vi "Trajectory_Execution_Dash_Write.vi"   [LabVIEW 2019]
uses:
  Trajectory_Execution_Globals.vi
  <vilib>/Rock Robotics/Network Tables/NT Write Number.vi
  <vilib>/Rock Robotics/Network Tables/NT Write Boolean.vi
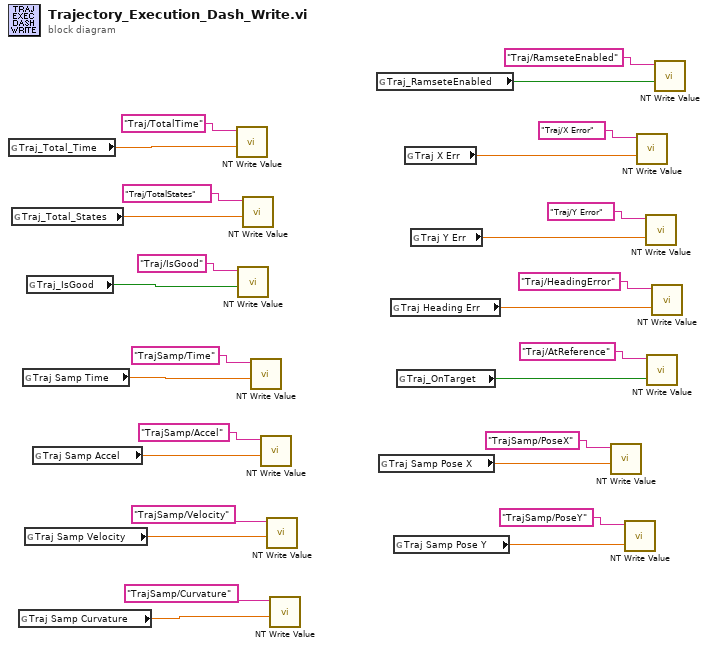
[diagram p0: block diagram]
diagram:
  n1 = global read "Trajectory_Execution_Globals.vi" "Traj_Total_Time"() -> (w14:dbl)
  n2 = global read "Trajectory_Execution_Globals.vi" "Traj_Total_States"() -> (w13:dbl)
  n3 = global read "Trajectory_Execution_Globals.vi" "Traj Samp Curvature"() -> (w8:dbl)
  n4 = global read "Trajectory_Execution_Globals.vi" "Traj Samp Time"() -> (w11:dbl)
  n5 = global read "Trajectory_Execution_Globals.vi" "Traj Samp Velocity"() -> (w9:dbl)
  n6 = global read "Trajectory_Execution_Globals.vi" "Traj_IsGood"() -> (w12:bool)
  n7 = global read "Trajectory_Execution_Globals.vi" "Traj Samp Accel"() -> (w10:dbl)
  n8 = call-poly <vilib>:"NT Write Value.vi"("Numeric"=w14, "Name"="Traj/TotalTime") -> ()  [unwired: 9 in, 1 out]
  n9 = call-poly <vilib>:"NT Write Value.vi"("Boolean"=w12, "Name"="Traj/IsGood") -> ()  [unwired: 9 in, 1 out]
  n10 = call-poly <vilib>:"NT Write Value.vi"("Numeric"=w13, "Name"="Traj/TotalStates") -> ()  [unwired: 9 in, 1 out]
  n11 = call-poly <vilib>:"NT Write Value.vi"("Numeric"=w11, "Name"="TrajSamp/Time") -> ()  [unwired: 9 in, 1 out]
  n12 = call-poly <vilib>:"NT Write Value.vi"("Numeric"=w10, "Name"="TrajSamp/Accel") -> ()  [unwired: 9 in, 1 out]
  n13 = call-poly <vilib>:"NT Write Value.vi"("Numeric"=w9, "Name"="TrajSamp/Velocity") -> ()  [unwired: 9 in, 1 out]
  n14 = call-poly <vilib>:"NT Write Value.vi"("Numeric"=w8, "Name"="TrajSamp/Curvature") -> ()  [unwired: 9 in, 1 out]
  n15 = global read "Trajectory_Execution_Globals.vi" "Traj_RamseteEnabled"() -> (w7:bool)
  n16 = global read "Trajectory_Execution_Globals.vi" "Traj Samp Pose X"() -> (w2:dbl)
  n17 = global read "Trajectory_Execution_Globals.vi" "Traj Heading Err"() -> (w4:dbl)
  n18 = global read "Trajectory_Execution_Globals.vi" "Traj Samp Pose Y"() -> (w1:dbl)
  n19 = global read "Trajectory_Execution_Globals.vi" "Traj_OnTarget"() -> (w3:bool)
  n20 = global read "Trajectory_Execution_Globals.vi" "Traj X Err"() -> (w6:dbl)
  n21 = global read "Trajectory_Execution_Globals.vi" "Traj Y Err"() -> (w5:dbl)
  n22 = call-poly <vilib>:"NT Write Value.vi"("Numeric"=w2, "Name"="TrajSamp/PoseX") -> ()  [unwired: 9 in, 1 out]
  n23 = call-poly <vilib>:"NT Write Value.vi"("Numeric"=w1, "Name"="TrajSamp/PoseY") -> ()  [unwired: 9 in, 1 out]
  n24 = call-poly <vilib>:"NT Write Value.vi"("Numeric"=w6, "Name"="Traj/X Error") -> ()  [unwired: 9 in, 1 out]
  n25 = call-poly <vilib>:"NT Write Value.vi"("Numeric"=w5, "Name"="Traj/Y Error") -> ()  [unwired: 9 in, 1 out]
  n26 = call-poly <vilib>:"NT Write Value.vi"("Boolean"=w3, "Name"="Traj/AtReference") -> ()  [unwired: 9 in, 1 out]
  n27 = call-poly <vilib>:"NT Write Value.vi"("Numeric"=w4, "Name"="Traj/HeadingError") -> ()  [unwired: 9 in, 1 out]
  n28 = call-poly <vilib>:"NT Write Value.vi"("Boolean"=w7, "Name"="Traj/RamseteEnabled") -> ()  [unwired: 9 in, 1 out]
